vi "Find Lines Array.vi"(6 "Ignore Index? (D=-1)":i32=-1, 8 "Ignore line? (D=-1)":i32=-1, 9 "Z":dbl, 10 "X":dbl, 11 "All Lines":T1) -> (0 "Distance to nearest":dbl, 1 "Index on Line":i32, 2 "Nearest Line":i32, 3 "Line found?":bool)   [LabVIEW 2014]
uses:
  Libraries/Map Data Folder/All-Lines.ctl
  Libraries/Map Data Folder/LineCluster.ctl
  Libraries/Map Data Folder/LineConnection.ctl
  Libraries/Map Data Folder/Map Data.lvlib
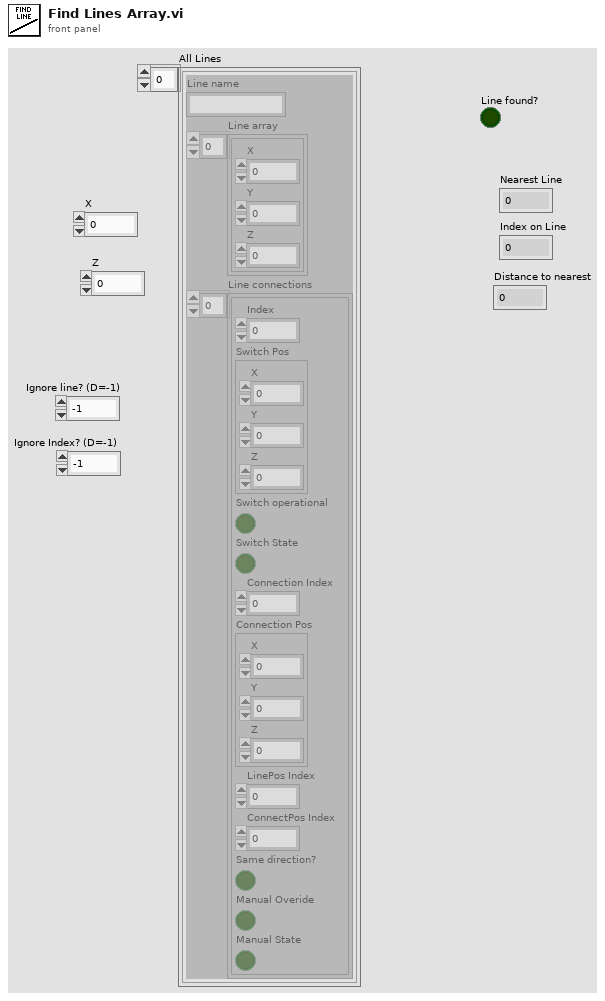
[diagram p1: front panel]
types:
  T1 = typedef "Map Data.lvlib/All-Lines.ctl" = T2[]
  T2 = typedef "Map Data.lvlib/LineCluster.ctl" = cluster{"Line name":string, "Line array":cluster{"X":dbl, "Y":dbl, "Z":dbl}[], "Line connections":T3[]}
  T3 = typedef "LineConnection.ctl" = cluster{"Index":i32, "Switch Pos":cluster{"X":dbl, "Y":dbl, "Z":dbl}, "Switch operational":bool, "Switch State":bool, "Connection Index":i32, "Connection Pos":cluster{"X":dbl, "Y":dbl, "Z":dbl}, "LinePos Index":i32, "ConnectPos Index":i32, "Same direction?":bool, "Manual Overide":bool, "Manual State":bool}
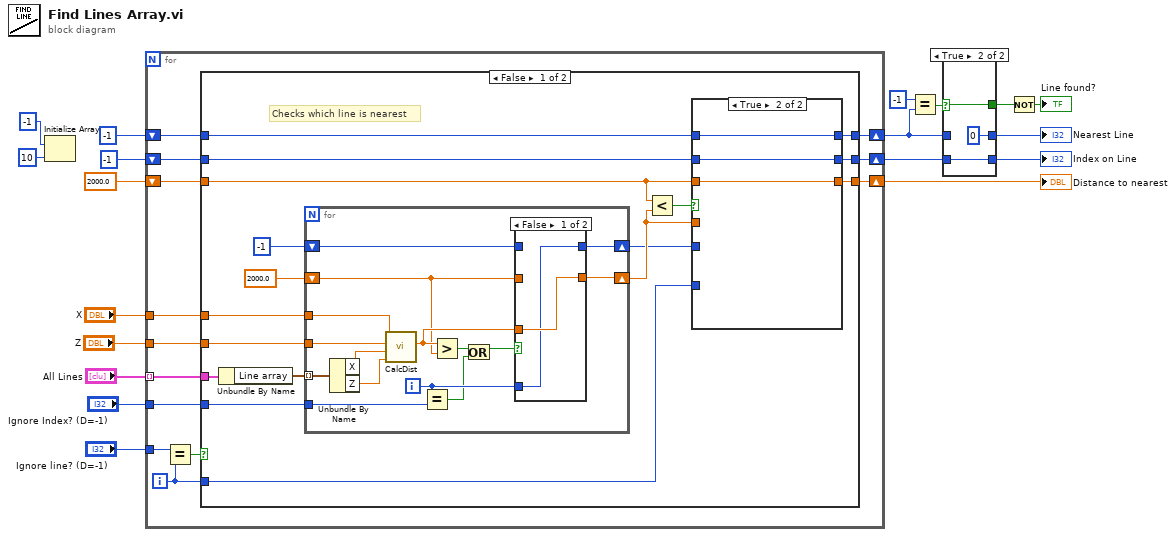
[diagram p0: block diagram]
diagram:
  n1 = Initialize Array(-1, 10 ("dimension size")) -> ()  [unwired: 1 out]
  n2 = for {
    tunnel: "All Lines" -> [w32] mode=indexing
    tunnel: "X" -> [w31]
    tunnel: "Z" -> [w30]
    shift-right: [w29] -> w17
    shift-left: 2000.0 ("Distance") -> [w26]
    shift-right: [w28] -> w5
    shift-left: -1 -> [w27]
    shift-right: [w24] -> w4
    shift-left: -1 -> [w25]
    tunnel: "Ignore line? (D=-1)" -> [w22]
    tunnel: "Ignore Index? (D=-1)" -> [w20]
    i -> [w23]
    n3 = Equal?(x=w22, y=w23) -> (x = y?=w21:bool)
    n4 = case shown="False" w21 {
      tunnel: w32 -> [w49 _]
      tunnel: w31 -> [w47 _]
      tunnel: w30 -> [w46 _]
      tunnel: [w44 w76] -> w29
      tunnel: [w43 w75] -> w28
      tunnel: w27 -> [w42 w75]
      tunnel: w26 -> [w41 w76]
      tunnel: w25 -> [w38 w77]
      tunnel: [w35 w77] -> w24
      tunnel: w23 -> [w34 _]
      tunnel: w20 -> [w33 _]
      frame False {
        # "Checks which line is nearest"
        n5 = Unbundle By Name(w49) -> ("Line array"=w48:cluster{"X":dbl, "Y":dbl, "Z":dbl}[])
        n6 = for {
          tunnel: w47 -> [w70]
          tunnel: w48 -> [w69] mode=indexing
          tunnel: w46 -> [w65]
          shift-right: [w62] -> w40
          shift-left: 2000.0 ("Distance") -> [w63]
          shift-right: [w60] -> w36
          shift-left: -1 -> [w61]
          tunnel: w33 -> [w58]
          i -> [w59]
          n7 = Unbundle By Name(w69) -> ("X"=w66:dbl, "Z"=w67:dbl)
          n8 = call "CalcDist.vi"("Y2"=w67, "X2"=w66, "Y1"=w65, "X1"=w70) -> ("Distance"=w64:dbl)  [unwired: 7 in]
          n9 = Equal?(x=w59, y=w58) -> (x = y?=w56:bool)
          n10 = Greater?(x=w64, y=w63) -> (0:w68:bool)
          n11 = Or(x=w68, y=w56) -> (x .or. y?=w57:bool)
          n12 = case shown="False" w57 {
            tunnel: w64 -> [w72 _]
            tunnel: [w72 w74] -> w62
            tunnel: w63 -> [_ w74]
            tunnel: w61 -> [_ w73]
            tunnel: w59 -> [w71 _]
            tunnel: [w71 w73] -> w60
            frame False {
            }
            frame True {
            }
          }
        }
        n13 = Less?(x=w41, y=w40) -> (x < y?=w39:bool)
        n14 = case shown="True" w39 {
          tunnel: w40 -> [w52 _]
          tunnel: [w52 w54] -> w44
          tunnel: w41 -> [_ w54]
          tunnel: w34 -> [w51 _]
          tunnel: [w51 w55] -> w43
          tunnel: w42 -> [_ w55]
          tunnel: w38 -> [_ w53]
          tunnel: w36 -> [w50 _]
          tunnel: [w50 w53] -> w35
          frame False {
          }
          frame True {
          }
        }
      }
      frame True {
      }
    }
  }
  "Distance to nearest" <- w17
  n15 = Equal?(x=-1, y=w5) -> (x = y?=w7:bool)
  n16 = case shown="True" w7 {
    selector: w7 -> [w78 w83]
    tunnel: [w78 w83] -> w8
    tunnel: w5 -> [w80 _]
    tunnel: [w80 0] -> w6
    tunnel: w4 -> [w79 w82]
    tunnel: [w79 w82] -> w3
    frame False {
    }
    frame True {
    }
  }
  "Nearest Line" <- w6
  "Index on Line" <- w3
  n17 = Not(x=w8) -> (.not. x?=→"Line found?":bool)
